vi "Generator.Synthesize Waveforms.vi"(4 "sweep index":i32=-1, 6 "Reset Phase?":bool, 8 "error in (no error)":errorcluster, 11 "Instrument.DAQ":refnum<class "Instrument.DAQ.lvclass">) -> (0 "error out":errorcluster, 3 "Instrument.DAQ":refnum<class "Instrument.DAQ.lvclass">)   [LabVIEW 2019, in "Instrument.DAQ.lvclass"]
uses:
  Instrument.DAQ.lvclass
  Instrument.DAQ.lvclass/Instrument.DAQ.ctl
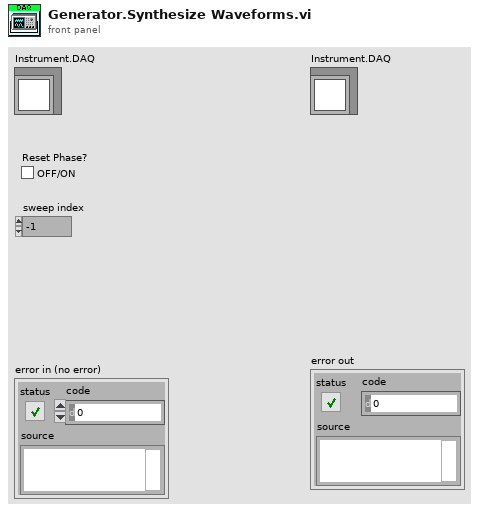
[diagram p1: front panel]
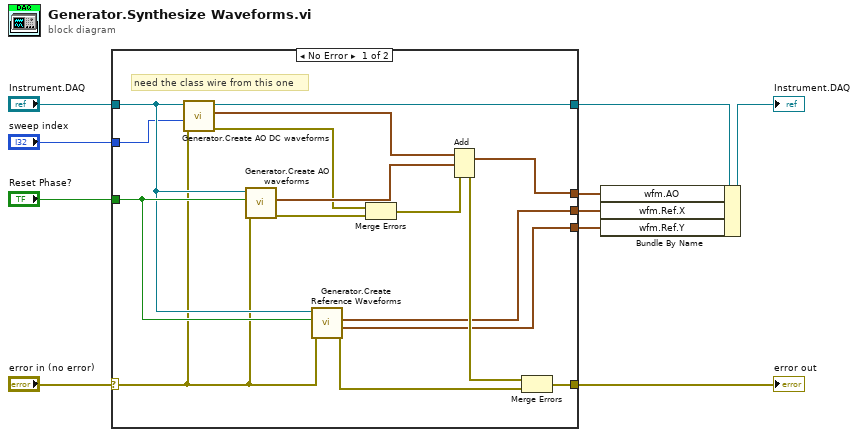
[diagram p0: block diagram]
diagram:
  n1 = case shown="No Error" "error in (no error)" {
    selector: "error in (no error)" -> [w23 w28]
    tunnel: [w11 _] -> w4
    tunnel: "Reset Phase?" -> [w26 _]
    tunnel: [w20 _] -> w2
    tunnel: [w25 w28] -> w9
    tunnel: "Instrument.DAQ" -> [w24 w27]
    tunnel: "sweep index" -> [w15 _]
    tunnel: [w21 w27] -> w3
    tunnel: [w12 _] -> w1
    frame No Error {
      # "need the class wire from this one"
      n2 = call "Generator.Create AO DC waveforms.vi"("error in (no error)"=w23, "sweep index"=w15, "Instrument.DAQ in"=w24) -> ("error out"=w16:errorcluster, "AO Array"=w19:waveform(dbl)[], "Instrument.DAQ out"=w21:refnum<class "Instrument.DAQ.lvclass">)  [unwired: 6 in]
      n3 = call "Generator.Create AO waveforms.vi"("error in (no error)"=w23, "reset phase"=w26, "Lockin.DAQ"=w24) -> ("error out"=w17:errorcluster, "AO Array"=w18:waveform(dbl)[])  [unwired: 6 in, 1 out]
      n4 = call "Generator.Create Reference Waveforms.vi"("error in (no error)"=w23, "reset phase"=w26, "Lockin.DAQ in"=w24) -> ("error out"=w22:errorcluster, "Y"=w12:waveform(dbl)[], "X"=w11:waveform(dbl)[])  [unwired: 5 in, 1 out]
      n5 = Merge Errors(w16, w17) -> (w14:errorcluster)
      n6 = Add(1:w18, 2:w19, 4:w14) -> (0:w20:waveform(dbl)[], 3:w13:errorcluster)
      n7 = Merge Errors(w13, w22) -> (w25:errorcluster)
    }
    frame Error {
    }
  }
  "error out" <- w9
  n8 = Bundle By Name(cluster=w3, "wfm.AO"=w2, "wfm.Ref.X"=w4, "wfm.Ref.Y"=w1) -> (→"Instrument.DAQ":refnum<class "Instrument.DAQ.lvclass">)
